vi "set group mapping info.vi"(7 "channel type":T1, 8 "error in (no error)":errorcluster, 10 "Map Info":variant, 11 "Item Ref in":T2 format="%.0x") -> (0 "error out":errorcluster, 3 "Item Ref out":T2 format="%.0x")   [LabVIEW 2016]
uses:
  <vilib>/NI Veristand/Custom Device API/Custom Device Item Ref.ctl
  SubVIs/Channel Type.ctl
  <vilib>/NI Veristand/Custom Device API/Set Item Property (Variant).vi
  <vilib>/NI VeriStand/Custom Device API/Custom Device API.lvlib
  FPGA Addon System Explorer.lvlib
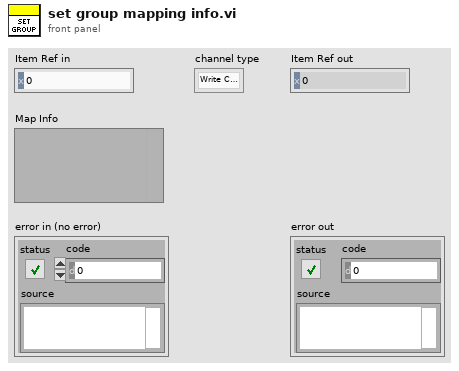
[diagram p1: front panel]
types:
  T1 = typedef "FPGA Addon System Explorer.lvlib/Channel Type.ctl" = enum16{"Write Channel", "Read Channel", "Write Waveform", "Read Waveform"}
  T2 = typedef "Custom Device API.lvlib/Custom Device Item Ref.ctl" = u64
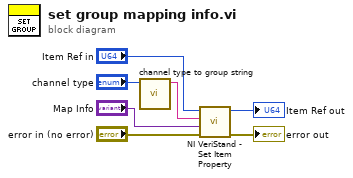
[diagram p0: block diagram]
diagram:
  n1 = call "channel type to group string.vi"("channel type"="channel type") -> ("FPGA.Controls"=w1:string)  [unwired: 10 in]
  n2 = call-poly <vilib>:"NI VeriStand - Set Item Property.vi"("error in (no error)"="error in (no error)", "Value"="Map Info", "Property Name"=w1, "Item Ref in"="Item Ref in") -> ("error out"=→"error out":errorcluster, "Item Ref out"=→"Item Ref out":T2)  [unwired: 5 in, 1 out]
